vi "Process Discovered Resources.vi"(9 "IO Resources in":T2[](array[typedef]), 10 "Software Resources in":T1[](array[typedef])) -> (1 "IO Resources out":T2[](array[typedef]), 2 "Software Resources out":T1[](array[typedef]), 5 "Is DAQmx installed?":bool)   [LabVIEW 2021, in "Acquisition.lvlib"]
doc: "Process the discovered resources and identify, correct, or drop entries as necessary."
uses:
  Acquisition.lvlib
  Host IO Resource.ctl
  Host Software Package.ctl
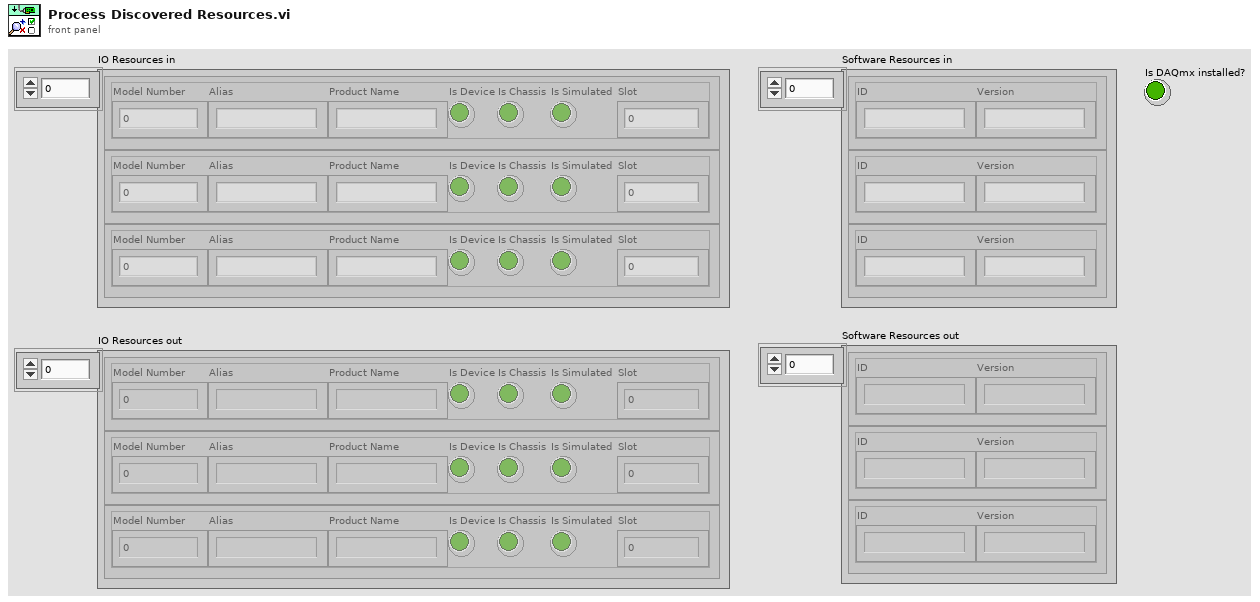
[diagram p1: front panel]
types:
  T1 = typedef "Acquisition.lvlib/Host Software Package.ctl" = cluster{"ID":string, "Version":string}
  T2 = typedef "Acquisition.lvlib/Host IO Resource.ctl" = cluster{"Model Number":u32, "Alias":string, "Product Name":string, "Is Device":bool, "Is Chassis":bool, "Is Simulated":bool, "Slot":i32}
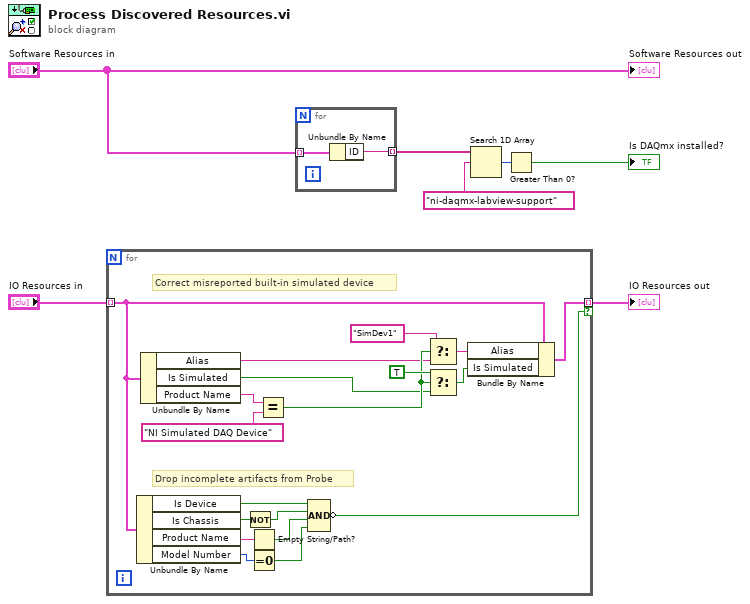
[diagram p0: block diagram]
diagram:
  n1 = for {
    tunnel: "IO Resources in" -> [w22] mode=indexing
    tunnel: [w26] -> w6 mode=indexing if=w14
    # "Correct misreported built-in simulated device"
    # "Drop incomplete artifacts from Probe"
    n2 = Unbundle By Name(w22) -> ("Is Device"=w18:bool, "Is Chassis"=w19:bool, "Product Name"=w21:string, "Model Number"=w20:u32)
    n3 = Unbundle By Name(w22) -> ("Alias"=w10:string, "Is Simulated"=w8:bool, "Product Name"=w9:string)
    n4 = Not(x=w19) -> (.not. x?=w15:bool)
    n5 = Empty String/Path?(string/path=w21) -> (empty?=w16:bool)
    n6 = Equal To 0?(x=w20) -> (x = 0?=w17:bool)
    n7 = Equal?(x=w9, y="NI Simulated DAQ Device") -> (x = y?=w11:bool)
    n8 = Compound Arithmetic op=AND(w18, w15, w16, w17) -> (invert w14:bool)
    n9 = Select(t="SimDev1", s=w11, f=w10) -> (s? t:f=w13:string)
    n10 = Select(t=TRUE, s=w11, f=w8) -> (s? t:f=w25:bool)
    n11 = Bundle By Name(cluster=w22, "Alias"=w13, "Is Simulated"=w25) -> (w26:T2)
  }
  "IO Resources out" <- w6
  n12 = for {
    tunnel: "Software Resources in" -> [w28] mode=indexing
    tunnel: [w27] -> w1 mode=indexing
    n13 = Unbundle By Name(w28) -> ("ID"=w27:string)
  }
  n14 = Search 1D Array(1D array=w1, element="ni-daqmx-labview-support") -> (index of element=w5:i32)  [unwired: 1 in]
  n15 = Greater Than 0?(x=w5) -> (x > 0?=→"Is DAQmx installed?":bool)
  "Software Resources out" <- "Software Resources in"
